vi "z.stack.run_grMD.vi"() -> ()   [LabVIEW 2012]
doc: "SciScan 1.2 160622"
uses:
  Custom Controls/experiment type.ctl
  <vilib>/Utility/VariantDataType/Type.ctl
  GFG/GFGnumericGet.vi
  GFG/GFGfpRefGet.vi
  GFG/GFGbooleanGet.vi
  GFG/GFG library.lvlib
  <vilib>/Utility/VariantDataType/VariantType.lvlib
panel:
  out "error out 2":errorcluster
  out "transposed array":dbl[][](array[numeric])
  out "data":dbl[][](array[numeric])
  in  "error in (no error)":errorcluster
  out "error out":errorcluster
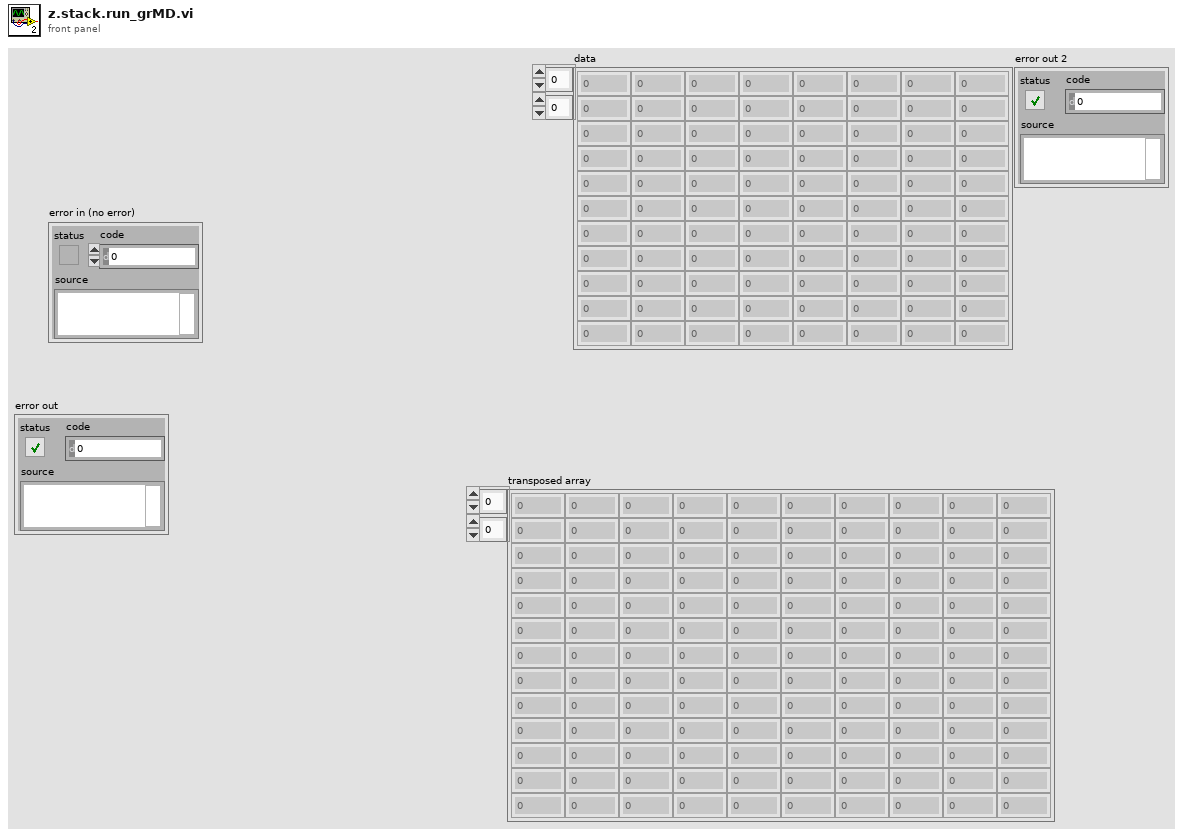
[diagram p1: front panel]
types:
  T1 = typedef "experiment type.ctl" = string
  T2 = enum8{"Enabled", "Disabled", "Disabled and Grayed Out"}
  T3 = cluster{"moveXabs":dbl, "moveYabs":dbl, "moveZabs":dbl}
  T4 = cluster{"WaveformChartRef":refnum<vi>, "DigitalRef":refnum<vi>, "ArrayRef":refnum<vi>, "TabControlRef":refnum<vi>, "EnumRef":refnum<vi>, "RingRef":refnum<vi>, "BooleanRef":refnum<vi>, "KnobRef":refnum<vi>, "SlideRef":refnum<vi>, "PathRef":refnum<vi>, "StringRef":refnum<vi>, "ComboBox":refnum<vi>, "WaveformGraphRef":refnum<vi>}
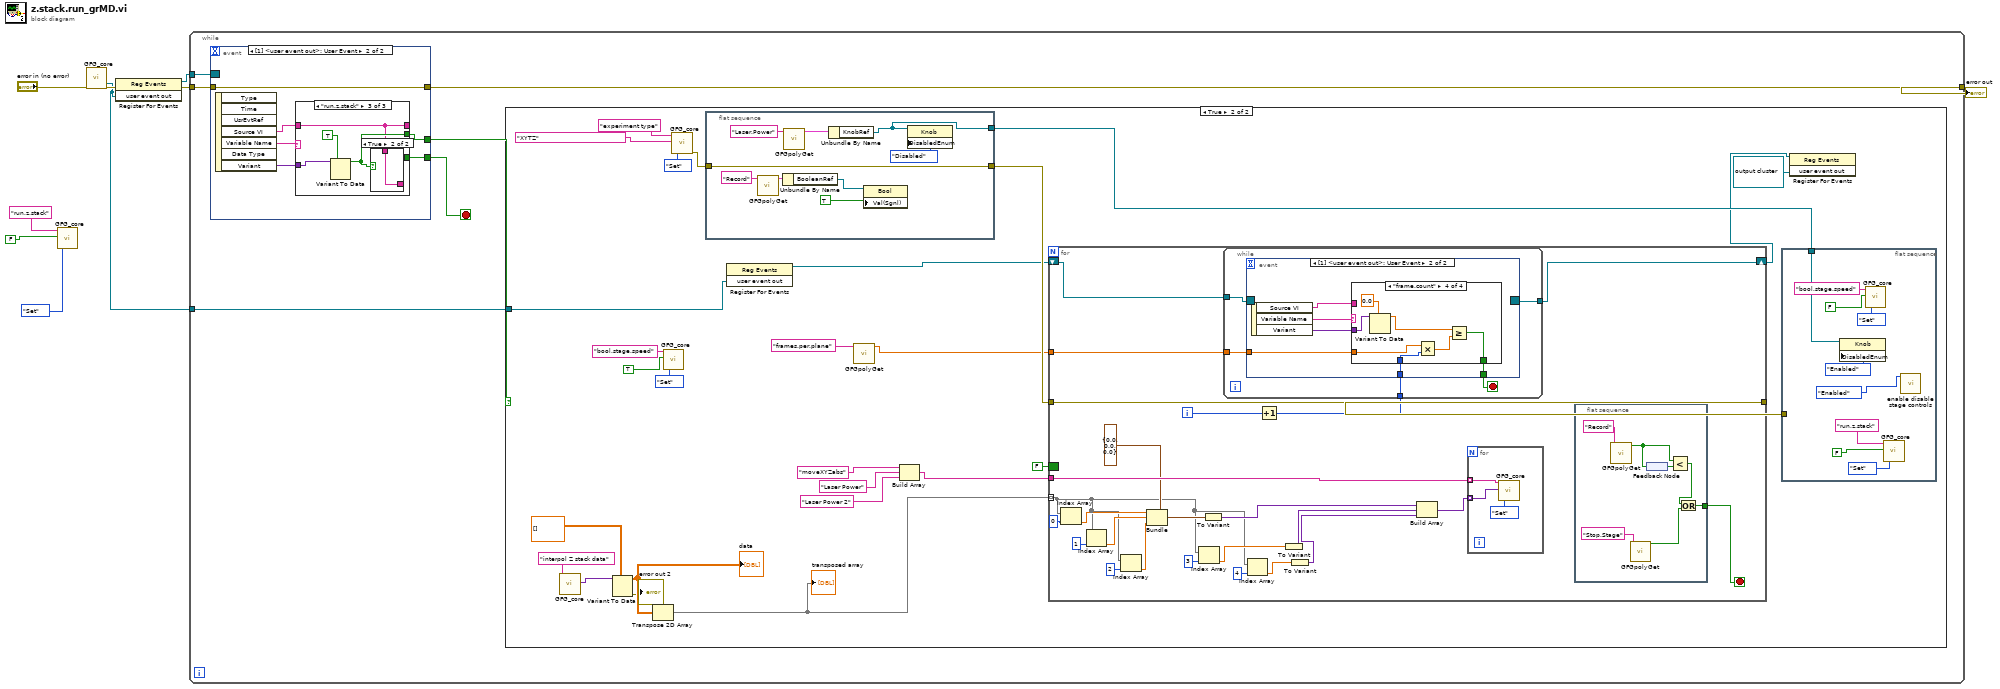
[diagram p0: block diagram]
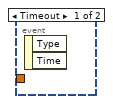
[diagram p3: hidden frame]
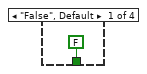
[diagram p4: hidden frame]
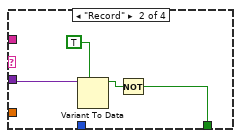
[diagram p5: hidden frame]
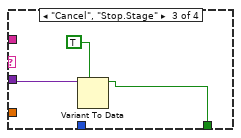
[diagram p6: hidden frame]
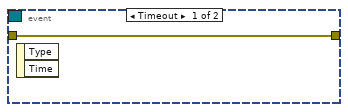
[diagram p7: hidden frame]
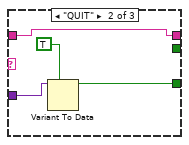
[diagram p9: hidden frame]
diagram:
  n1 = call "GFG_core.vi"("Variable Name in"="run.z.stack", "Variant in"=FALSE, "Action"=enum16{"Init", "Set", "Get"}."Set") -> ()  [unwired: 10 in, 7 out]
  n2 = call "GFG_core.vi"("error in (no error)"="error in (no error)") -> ("user event out"=w1:refnum<user-event>, "error out"=w6:errorcluster)  [unwired: 12 in, 5 out]
  n3 = register-events(error in=w6, w1) -> (reference out=w5:refnum<event-registration>, error out=w8:errorcluster)  [unwired: 1 in]
  n4 = while {
    tunnel: w5 -> [w15]
    tunnel: w8 -> [w14]
    tunnel: [w13] -> w9
    tunnel: w1 -> [w10]
    stop <- w12 stop-if-true
    n5 = event shown="[1] <user event out>: User Event" {
      selector: w15 -> [_ _]
      dyn-events: _ -> [_ _]
      timeout: _ -> [_ _]
      tunnel: w14 -> [w122 w128]
      tunnel: [w122 w128] -> w13
      tunnel: [_ w125] -> w12
      tunnel: [_ w124] -> w11
      event Timeout {
        n6 = event-data() -> ()  [unwired: 1 in, 2 out]
      }
      event User Event {
        n7 = event-data() -> ("Source VI"=w123:string, "Variable Name"=w127:string, "Variant"=w126:variant)  [unwired: 1 in, 4 out]
        n8 = case shown="\"run.z.stack\"" w127 {
          tunnel: w126 -> [_ w132 w136]
          tunnel: [_ w131 _] -> w125
          tunnel: [_ _ w135] -> w124
          tunnel: w123 -> [w129 w130 w134]
          tunnel: [w129 w130 w134] -> _
          frame "False", Default {
          }
          frame "QUIT" {
            n9 = Variant To Data(type=TRUE, Variant=w132) -> (data=w131:bool)  [unwired: 1 in, 1 out]
          }
          frame "run.z.stack" {
            n10 = Variant To Data(type=TRUE, Variant=w136) -> (data=w135:bool)  [unwired: 1 in, 1 out]
            n11 = case shown="True" w135 {
              tunnel: w134 -> [_ w138]
              tunnel: [_ w138] -> _
              frame False {
              }
              frame True {
              }
            }
          }
        }
      }
    }
    n12 = case shown="True" w11 {
      tunnel: w10 -> [_ w17]
      frame False {
      }
      frame True {
        n13 = call "GFG_core.vi"("Variable Name in"="interpol Z stack data") -> ("Variant Out"=w40:variant)  [unwired: 12 in, 6 out]
        n14 = Variant To Data(type=dbl[][] [] ("Interpolated Data"), Variant=w40) -> (data=w38:dbl[][], error out=→"error out 2":errorcluster)  [unwired: 1 in]
        "data" <- w38
        n15 = Transpose 2D Array(2D array=w38) -> (transposed array=w37:dbl[][])
        "transposed array" <- w37
        n16 = call "GFG_core.vi"("Variable Name in"="bool.stage.speed", "Variant in"=TRUE, "Action"=enum16{"Init", "Set", "Get"}."Set") -> ()  [unwired: 10 in, 7 out]
        n17 = call "GFG_core.vi"("Variable Name in"="experiment type", "Variant in"=T1 "XYTZ" ("experiment type"), "Action"=enum16{"Init", "Set", "Get"}."Set") -> ("error out"=w31:errorcluster)  [unwired: 10 in, 6 out]
        n18 = flat-sequence {
          tunnel: w31 -> [w50]
          tunnel: [w50] -> w32
          tunnel: [w43] -> w29
          frame #0 {
            n19 = call-poly "GFGpolyGet.vi"("Variable Name in"="Record") -> ("output cluster"=w49:T4)  [unwired: 9 in, 1 out]
            n20 = Unbundle By Name(w49) -> ("BooleanRef"=w48:refnum<vi>)
            n21 = call-poly "GFGpolyGet.vi"("Variable Name in"="Laser.Power") -> ("output cluster"=w45:T4)  [unwired: 9 in, 1 out]
            n22 = Unbundle By Name(w45) -> ("KnobRef"=w43:refnum<vi>)
            n23 = property class="Bool"(reference=w48, "Val(Sgnl)"=TRUE) -> ()  [unwired: 1 in, 2 out]
            n24 = property class="Knob"(reference=w43, "DisabledEnum"=T2."Disabled" ("Disabled")) -> ()  [unwired: 1 in, 2 out]
          }
        }
        n25 = register-events(w17) -> (reference out=w18:refnum<event-registration>)  [unwired: 2 in, 1 out]
        n26 = call-poly "GFGpolyGet.vi"("Variable Name in"="frames.per.plane") -> ("Numeric"=w24:dbl)  [unwired: 8 in, 2 out]
        n27 = Build Array("moveXYZabs" ("Variable Name in"), "Laser Power" ("Variable Name in"), "Laser Power 2" ("Variable Name in")) -> (w25:string[])
        n28 = for {
          tunnel: w37 -> [w68] mode=indexing
          tunnel: w25 -> [w85]
          tunnel: w32 -> [w64]
          tunnel: [w64] -> w33
          tunnel: w24 -> [w66]
          shift-right: [w63] -> w19
          shift-left: w18 -> [w62]
          border: FALSE ("Boolean Value OUT") -> [_]
          i -> [w65]
          stop <- w84 stop-if-true
          n29 = Index Array(array=w68, index=0) -> (element=w70:dbl)
          n30 = Index Array(array=w68, index=1) -> (element=w71:dbl)
          n31 = Index Array(array=w68, index=2) -> (element=w74:dbl)
          n32 = Bundle(cluster=T3 {"moveXabs"=0.0, "moveYabs"=0.0, "moveZabs"=0.0} ("output cluster"), "moveXabs"=w70, "moveYabs"=w71, "moveZabs"=w74) -> (w79:T3)
          n33 = Index Array(array=w68, index=3) -> (element=w78:dbl)
          n34 = To Variant(anything=w79) -> (Variant=w80:variant)
          n35 = Index Array(array=w68, index=4) -> (element=w77:dbl)
          n36 = Increment(x=w65) -> (x+1=w61:i32)
          n37 = while {
            tunnel: w62 -> [w90]
            tunnel: w66 -> [w89]
            tunnel: w61 -> [w88]
            tunnel: [w86] -> w63
            stop <- w87 stop-if-true
            n38 = event shown="[1] <user event out>: User Event" {
              selector: w90 -> [_ _]
              dyn-events: [_ _] -> w86
              timeout: _ -> [_ _]
              tunnel: w89 -> [_ w94]
              tunnel: w88 -> [_ w93]
              tunnel: [_ w92] -> w87
              event Timeout {
                n39 = event-data() -> ()  [unwired: 1 in, 2 out]
              }
              event User Event {
                n40 = event-data() -> ("Source VI"=w91:string, "Variable Name"=w96:string, "Variant"=w95:variant)  [unwired: 1 in]
                n41 = case shown="\"frame.count\"" w96 {
                  tunnel: w95 -> [_ w100 w103 w111]
                  tunnel: w94 -> [_ _ _ w109]
                  tunnel: w93 -> [_ _ _ w108]
                  tunnel: [FALSE w98 w102 w105] -> w92
                  tunnel: w91 -> [_ _ _ _]
                  frame "False", Default {
                  }
                  frame "Record" {
                    n42 = Variant To Data(type=TRUE, Variant=w100) -> (data=w99:bool)  [unwired: 1 in, 1 out]
                    n43 = Not(x=w99) -> (.not. x?=w98:bool)
                  }
                  frame "Cancel", "Stop.Stage" {
                    n44 = Variant To Data(type=TRUE, Variant=w103) -> (data=w102:bool)  [unwired: 1 in, 1 out]
                  }
                  frame "frame.count" {
                    n45 = Variant To Data(type=0.0, Variant=w111) -> (data=w106:dbl)  [unwired: 1 in, 1 out]
                    n46 = Multiply(x=w109, y=w108) -> (x*y=w107:dbl)
                    n47 = Greater Or Equal?(x=w106, y=w107) -> (x >= y?=w105:bool)
                  }
                }
              }
            }
          }
          n48 = To Variant(anything=w78) -> (Variant=w81:variant)
          n49 = To Variant(anything=w77) -> (Variant=w82:variant)
          n50 = Build Array(w80, w81, w82) -> (w67:variant[])
          n51 = for {
            tunnel: w67 -> [w120] mode=indexing
            tunnel: w85 -> [w121] mode=indexing
            n52 = call "GFG_core.vi"("Variable Name in"=w121, "Variant in"=w120, "Action"=enum16{"Init", "Set", "Get"}."Set") -> ()  [unwired: 10 in, 7 out]
          }
          n53 = flat-sequence {
            tunnel: [w115] -> w84
            frame #0 {
              n54 = call-poly "GFGpolyGet.vi"("Variable Name in"="Record") -> ("Boolean Value OUT"=w114:bool)  [unwired: 9 in, 1 out]
              n55 = call-poly "GFGpolyGet.vi"("Variable Name in"="Stop.Stage") -> ("Boolean Value OUT"=w116:bool)  [unwired: 9 in, 1 out]
              n56 = feedback-in #1(w114) -> ()
              n57 = feedback #1() -> (w113:bool)
              n58 = Less?(x=w114, y=w113) -> (x < y?=w112:bool)
              n59 = Or(x=w112, y=w116) -> (x .or. y?=w115:bool)
            }
          }
        }
        n60 = flat-sequence {
          tunnel: w33 -> [_]
          tunnel: w29 -> [w55]
          frame #0 {
            n61 = property class="Knob"(reference=w55, "DisabledEnum"=T2."Enabled" ("Disabled")) -> ()  [unwired: 1 in, 2 out]
            n62 = call "GFG_core.vi"("Variable Name in"="bool.stage.speed", "Variant in"=FALSE, "Action"=enum16{"Init", "Set", "Get"}."Set") -> ()  [unwired: 10 in, 7 out]
            n63 = call "GFG_core.vi"("Variable Name in"="run.z.stack", "Variant in"=FALSE, "Action"=enum16{"Init", "Set", "Get"}."Set") -> ()  [unwired: 10 in, 7 out]
            n64 = call "enable disable stage controls.vi"("Disabled"=T2."Enabled") -> ()  [unwired: 11 in]
          }
        }
        n65 = register-events(reference=w19, refnum<user-event> refnum ("event source")) -> ()  [unwired: 1 in, 2 out]
      }
    }
  }
  "error out" <- w9
